vi "Start Cooker.vi"(8 "error in (no error)":errorcluster, 9 "Duration (s)":dbl, 10 "Set Fire (%)":dbl min=0.0 max=100.0 format="%.2f %", 11 "Direct Cooker in":refnum<class "Direct Cooker.lvclass">) -> (0 "error out":errorcluster, 3 "Direct Cooker out":refnum<class "Direct Cooker.lvclass">)   [LabVIEW 2024, in "Cooker Actor.lvlib" / "Direct Cooker.lvclass"]
uses:
  Direct Cooker.lvclass
  C:/Program Files/National Instruments/LabVIEW 2024/vi.lib/ActorFramework/Actor/Actor.lvclass
  Cooker Actor Messages/Update Kitchen Fire and Timer Msg/Update Kitchen Fire and Timer Msg.lvclass
  C:/Program Files/National Instruments/LabVIEW 2024/vi.lib/ActorFramework/Message/Message.lvclass
  <vilib>/ActorFramework/Actor/Actor.lvclass/Actor.ctl
  <vilib>/ActorFramework/Message Enqueuer/Message Enqueuer.lvclass/Message Enqueuer.ctl
  <vilib>/ActorFramework/Message Enqueuer/Init from Existing Queue.vi
  <vilib>/ActorFramework/Message Enqueuer/Message Enqueuer.lvclass
  Direct Cooker.lvclass/Direct Cooker.ctl
  <vilib>/ActorFramework/Actor/Actor.lvclass
  C:/Users/burakkorkmaz/Desktop/Leveling/repo/Cooker Actor/Cooker Actor Messages/Update Kitchen Fire and Timer Msg/Update Kitchen Fire and Timer Msg.lvclass
  C:/Users/burakkorkmaz/Desktop/Leveling/repo/Cooker Actor/Cooker Actor/Cooker Actor.lvclass
  C:/Users/burakkorkmaz/Desktop/Leveling/repo/Cooker Actor/Direct Cooker/Direct Cooker.lvclass
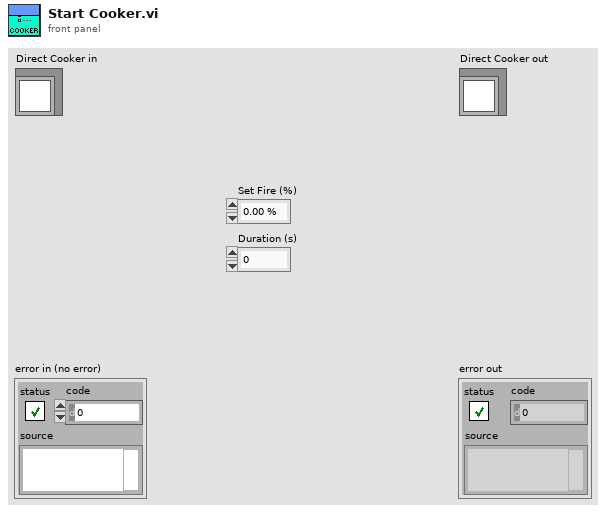
[diagram p1: front panel]
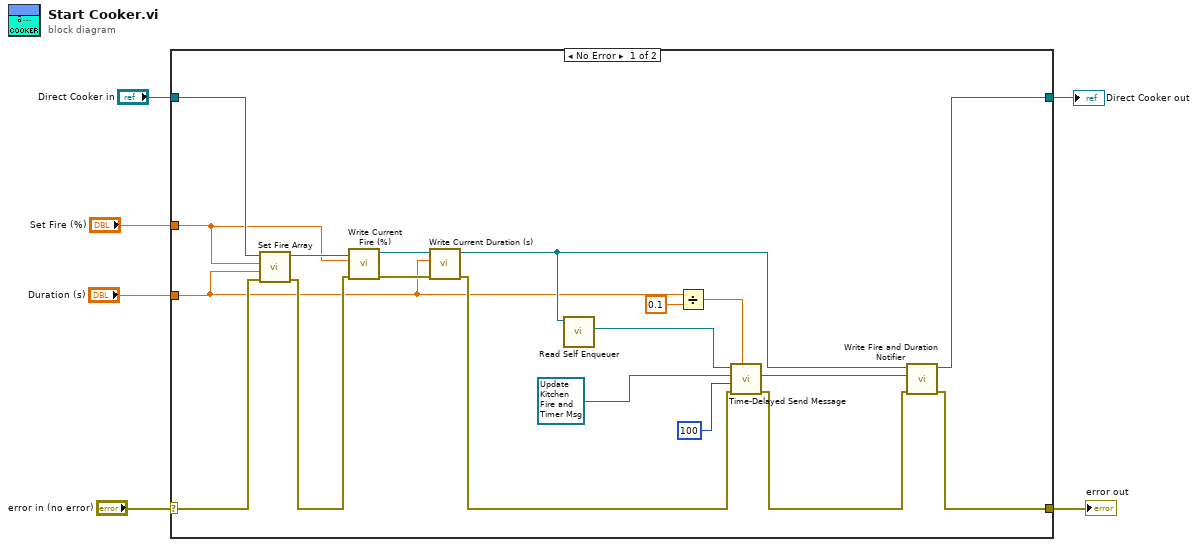
[diagram p0: block diagram]
diagram:
  n1 = case shown="No Error" "error in (no error)" {
    selector: "error in (no error)" -> [w24 w26]
    tunnel: [w16 w26] -> w5
    tunnel: "Direct Cooker in" -> [w25 w27]
    tunnel: [w19 w27] -> w3
    tunnel: "Set Fire (%)" -> [w8 _]
    tunnel: "Duration (s)" -> [w7 _]
    frame No Error {
      n2 = call-dynamic "Set Fire Array.vi"("error in (no error)"=w24, "Duration (s)"=w7, "Fire (%)"=w8, "Cooker Actor in"=w25) -> ("error out"=w12:errorcluster, "Cooker Actor out"=w10:refnum<class "Direct Cooker.lvclass">)  [unwired: 6 in]
      n3 = call-dynamic "Write Current Fire (%).vi"("error in (no error)"=w12, "Current Fire (%)"=w8, "Cooker Actor in"=w10) -> ("error out"=w14:errorcluster, "Cooker Actor out"=w13:refnum<class "Direct Cooker.lvclass">)  [unwired: 7 in]
      n4 = call-dynamic "Write Current Duration (s).vi"("error in (no error)"=w14, "Current Duration (s)"=w7, "Cooker Actor in"=w13) -> ("error out"=w11:errorcluster, "Cooker Actor out"=w9:refnum<class "Direct Cooker.lvclass">)  [unwired: 7 in]
      n5 = call <vilib>:"Read Self Enqueuer.vi"("Actor"=w9) -> ("Self Enqueuer"=w22:refnum<class "Message Enqueuer.lvclass">)  [unwired: 10 in]
      n6 = Divide(x=w7, y=0.1) -> (x/y=w21:dbl)
      n7 = call <vilib>:"Time-Delayed Send Message.vi"("# Copies (0 = infinite repeat)"=w21, "error in (no error)"=w11, "Milliseconds To Wait"=100, "Message"=refnum<class "Update Kitchen Fire and Timer Msg.lvclass"> refnum ("Cooker Actor.lvlib:Update Kitchen Fire and Timer Msg.lvclass"), "Message Enqueuer"=w22) -> ("error out"=w17:errorcluster, "Delivery Notifier"=w18:refnum<notifier>)  [unwired: 5 in]
      n8 = call-dynamic "Write Fire and Duration Notifier.vi"("error in (no error)"=w17, "Fire and Duration Notifier"=w18, "Cooker Actor in"=w9) -> ("error out"=w16:errorcluster, "Cooker Actor out"=w19:refnum<class "Direct Cooker.lvclass">)  [unwired: 7 in]
    }
    frame Error {
    }
  }
  "error out" <- w5
  "Direct Cooker out" <- w3
